vi "Stop Core.vi"(10 "final error code":i32, 11 "Network Endpoint in":refnum<class "Network Endpoint.lvclass">) -> (3 "Network Endpoint out":refnum<class "Network Endpoint.lvclass">)   [LabVIEW 2020, in "Network Endpoint.lvlib" / "Network Endpoint.lvclass"]
doc: "Defines what the actor does before it stops. Use the <B>final error code</B> input to determine whether the actor shut down normally. By default, a value of 43 indicates the actor stopped normally. Any other value indicates the actor stopped due to an error. However, descendants of Actor.lvclass can override Actor.lvclass:Handle Error.vi to change this behavior.\n\nBy default, this method does nothing. A descendant class may override it to define behavior, such as shutting down any processes the actor initiated in its override of Actor.lvclass:Actor Core.vi."
uses:
  Network Endpoint.lvclass
  Network Endpoint.lvclass/Network Endpoint.ctl
  Cache Manager/Cache Manager.lvclass/Cache Manager.ctl
  <vilib>/ActorFramework/Actor/Actor.lvclass
  Abstract Classes/Message Stream/Message Stream.lvclass
  Cache Manager/Cache Manager.lvclass
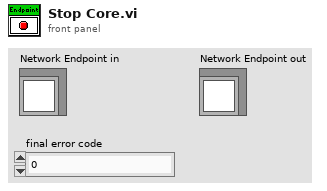
[diagram p1: front panel]
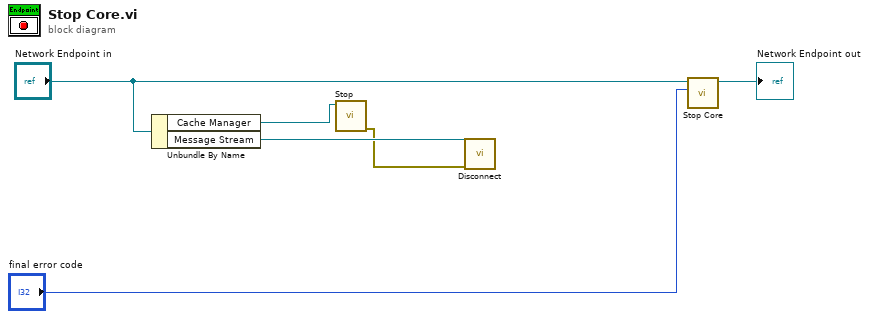
[diagram p0: block diagram]
diagram:
  n1 = Unbundle By Name("Network Endpoint in") -> ("Cache Manager"=w2:refnum<class "Cache Manager.lvclass">, "Message Stream"=w3:refnum<class "Message Stream.lvclass">)
  n2 = call "Stop.vi"("Cache Manager DVR in"=w2) -> ("error out"=w1:errorcluster)  [unwired: 9 in, 1 out]
  n3 = call-dynamic "Disconnect.vi"("error in (no error)"=w1, "Message Stream in"=w3) -> ()  [unwired: 8 in, 2 out]
  n4 = call-parent "Stop Core.vi"("final error code"="final error code", "Actor in"="Network Endpoint in") -> ("Actor out"=→"Network Endpoint out":refnum<class "Network Endpoint.lvclass">)  [unwired: 9 in]
